vi "Analog Output - N Channels - N Samples.vi"() -> ()   [LabVIEW 2019]
uses:
  <vilib>/myRIO/Common/Instrument Driver Framework/ELVIS III v1.0/AO Block/vis/ELVIS III v1.0 Close AO Block.vi
  <vilib>/myRIO/Common/Instrument Driver Framework/myRIO v1.0/UART/vis/myRIO v1.0 Close UART.vi
  <vilib>/myRIO/Common/Instrument Driver Framework/ELVIS III v1.0/AO Block/vis/ELVIS III v1.0 Unreserve AO Block.vi
  <vilib>/myRIO/Common/Instrument Driver Framework/ELVIS III v1.0/AO Block/vis/ELVIS III v1.0 Build MUX Configuration AO Block.vi
  <vilib>/Utility/error.llb/Error Cluster From Error Code.vi
  <vilib>/myRIO/Common/Instrument Driver Framework/ELVIS III v1.0/AO Block/vis/ELVIS III v1.0 AO Block Write.vi
  <vilib>/myRIO/Common/Instrument Driver Framework/ELVIS III v1.0/Resource Manager/vis/ELVIS III v1.0 Unreserve Channel List.vi
  <vilib>/myRIO/Common/Instrument Driver Framework/myRIO v1.0/myRIO v1.0 Close.vi
  <vilib>/myRIO/Common/Instrument Driver Framework/Utilities/vis/FPGA Ref Manager.vi
  <vilib>/myRIO/Common/Instrument Driver Framework/ELVIS III v1.0/ELVIS III v1.0 Reset FPGA.vi
  <vilib>/myRIO/Common/Instrument Driver Framework/myRIO v1.0/IRQ/vis/myRIO v1.0 IRQ Info FGV.vi
  <vilib>/myRIO/Common/Instrument Driver Framework/myRIO v1.0/IRQ/vis/myRIO v1.0 Timer IRQ Info FGV.vi
  <vilib>/myRIO/Common/Instrument Driver Framework/myRIO v1.0/IRQ/vis/myRIO v1.0 ISR Agent.vi
  <vilib>/myRIO/Instrument Drivers/Utilities/vis/Reset Index.vi
  <vilib>/myRIO/Common/Instrument Driver Framework/myRIO v1.0/Resource Manager/vis/myRIO v1.0 Block Write Resource Manager.vi
  <vilib>/myRIO/Instrument Drivers/Utilities/Utilities.lvlib
  <vilib>/myRIO/Instrument Drivers/Onboard IO/AO Block/AO Block.lvlib
panel:
  in  "Generate Waveform":bool
  in  "AO1 - Triangle Frequency (Hz)":dbl=10.0 format="%#_13g"
  in  "AO1 - Triangle Amplitude (V)":dbl=5.0 min=-10.0 max=10.0 step=0.1 format="%#_13g"
  in  "AO0 - Sine Frequency (Hz)":dbl=10.0 format="%#_13g"
  in  "AO0 - Sine Amplitude (V)":dbl=5.0 min=-10.0 max=10.0 step=0.1 format="%#_13g"
  in  "Stop":bool
  # "ELVIS III Control IO"
  # "模拟输出N通道"
  # "Overview: Outputs one period of Sine and Triangle waves on Bank A, Channels AO0 and AO1 (A/AO0 and A/AO1).\nInstructions:\n1. Configure the sine wave and triangle wave properties below.\n2. Connect A/AO0 to the positive lead of a load, and connect AGND to the negative lead of the load. Connect A/AO1 to the positive lead of another load, and connect AGND to the negative lead of the corresponding load. AGND is the ground reference terminal for analog output channels.\n3. Run the VI.\n4. Modify the Amplitude and Frequency controls to change the sine and triangle waves.\n5. Press Generate Waveform to output the sine and triangle waves."
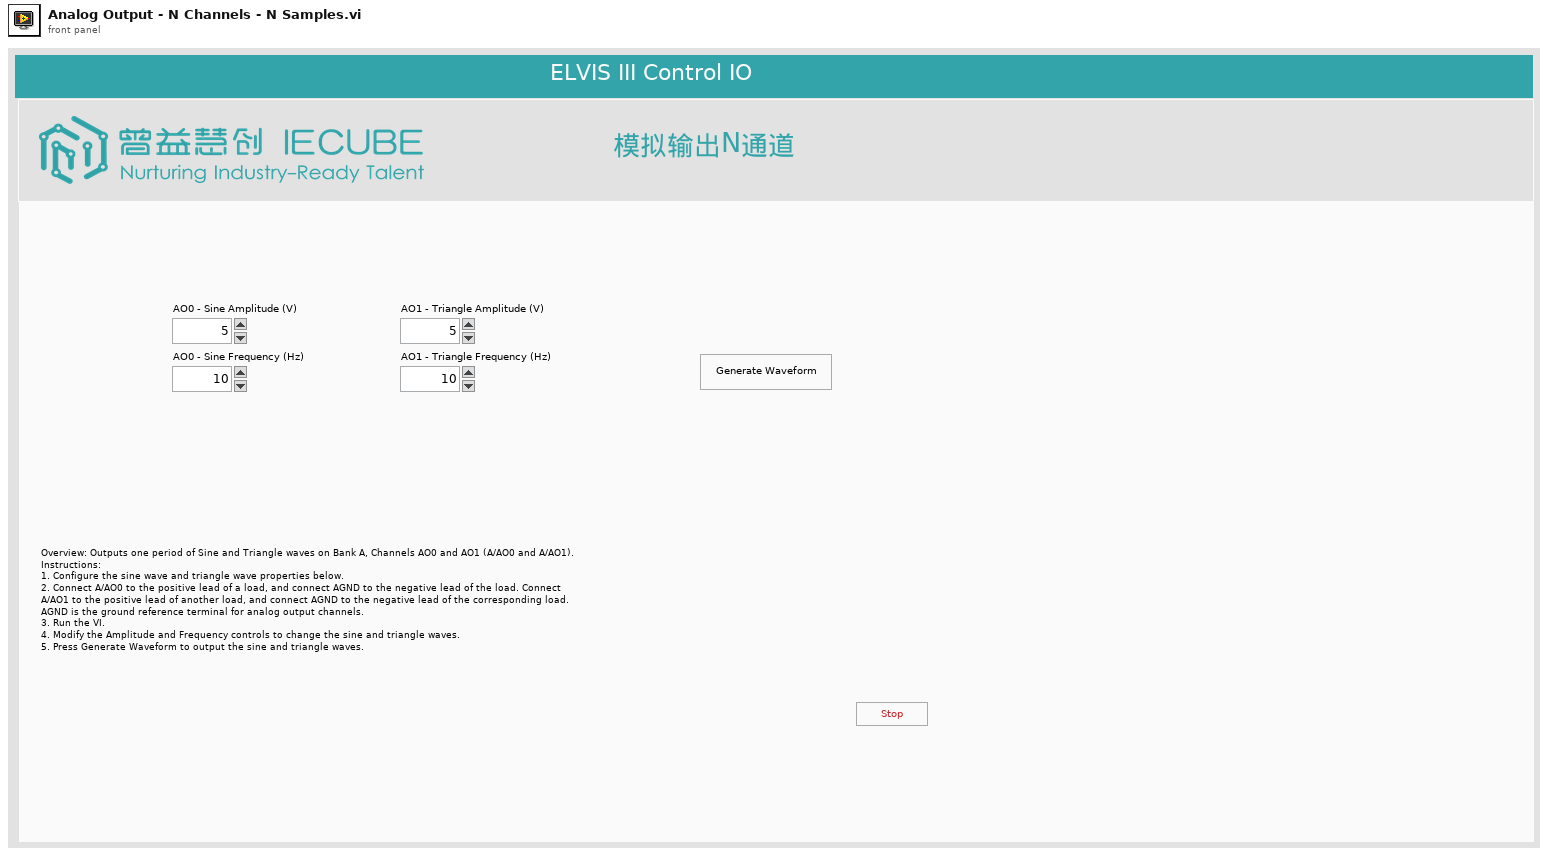
[diagram p1: front panel]
types:
  T1 = typedef "AO Block.lvlib/AO Block Reference.ctl" = cluster{"myRIO Reference":T2, "AO (N Samples) Channels List":T6, "AO (N Samples) Scaling Constants List":T8[]}
  T2 = typedef "myRIO Generic Hardware Reference.ctl" = cluster{"myRIO Model":T3, "myRIO Hardware Reference":T4}
  T3 = typedef "Hardware Version Enum.ctl" = enum16{"Unknown", "myRIO-1900", "myRIO-1950", "roboRIO", "NI ELVIS RIO CM", "ELVIS III"}
  T4 = typedef "myRIO v1.0 Reference.ctl" = cluster{"Generic FPGA Reference":T5, "Allow multiple opens":bool}
  T5 = typedef "Generic FPGA Reference.ctl" = refnum<k20>
  T6 = typedef "AO Block Channels List.ctl" = T7[]
  T7 = typedef "AO Block Channels Enum.ctl" = enum16{"Not Connected", "A/AO0 (N Samples)", "A/AO1 (N Samples)", "B/AO0 (N Samples)", "B/AO1 (N Samples)"}
  T8 = typedef "Analog Scaling Constants.ctl" = cluster{"LSB Weight (Volts)":dbl, "Offset (Volts)":dbl, "Signed?":bool}
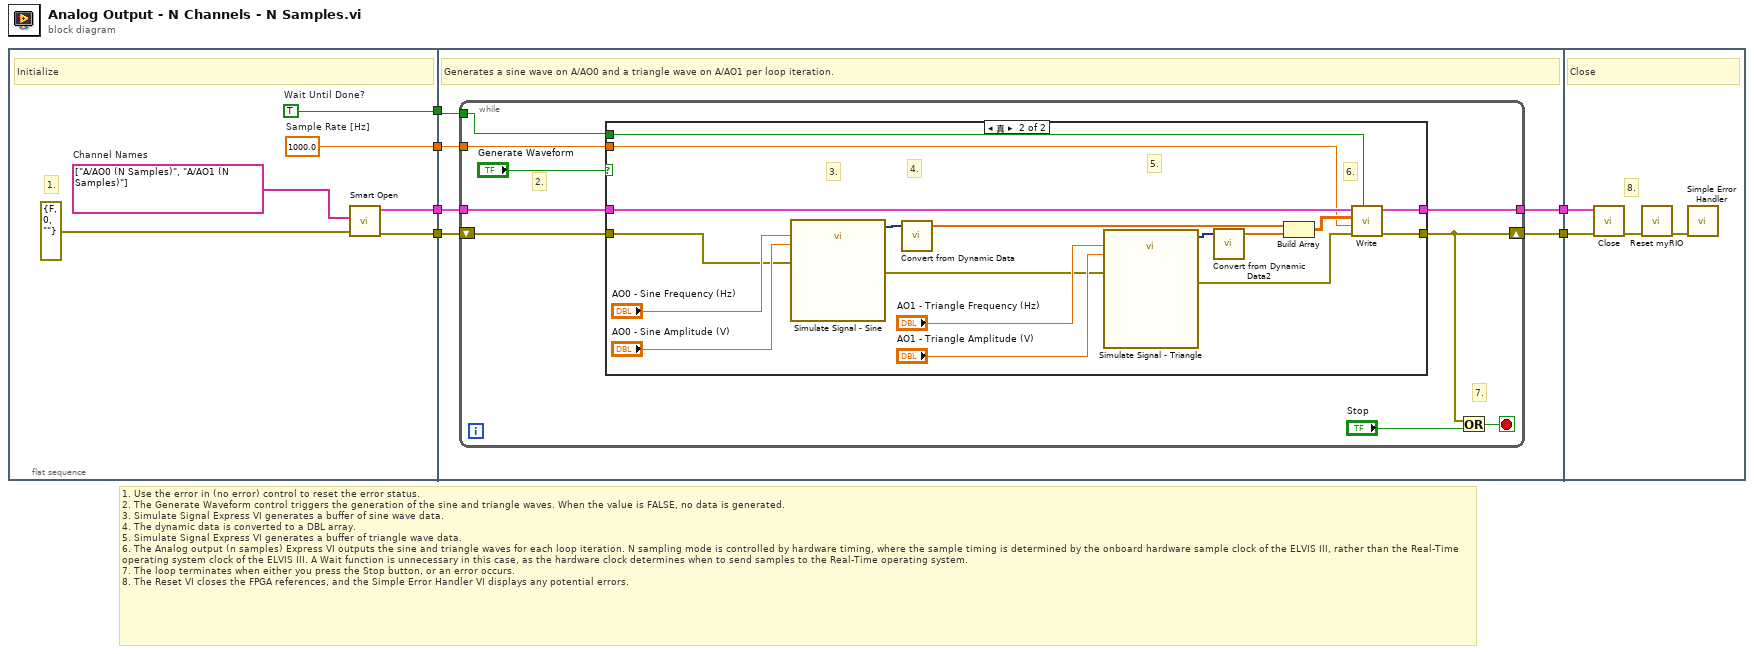
[diagram p0: block diagram]
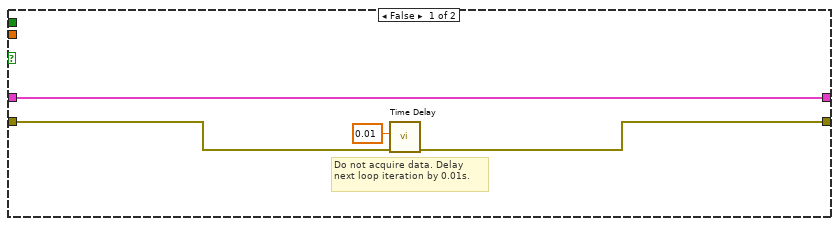
[diagram p2: hidden frame]
diagram:
  # "1. Use the error in (no error) control to reset the error status.\n2. The Generate Waveform control triggers the generation of the sine and triangle waves. When the value is FALSE, no data is generated.\n3. Simulate Signal Express VI generates a buffer of sine wave data.\n4. The dynamic data is converted to a DBL array.\n5. Simulate Signal Express VI generates a buffer of triangle wave data.\n6. The Analog output (n samples) Express VI outputs the sine and triangle waves for each loop iteration. N sampling mode is controlled by hardware timing, where the sample timing is determined by the onboard hardware sample clock of the ELVIS III, rather than the Real-Time operating system clock of the ELVIS III. A Wait function is unnecessary in this case, as the hardware clock determines when to send samples to the Real-Time operating system.\n7. The loop terminates when either you press the Stop button, or an error occurs.\n8. The Reset VI closes the FPGA references, and the Simple Error Handler VI displays any potential errors."
  n1 = flat-sequence {
    tunnel: [w10] -> w5
    tunnel: [w9] -> w4
    tunnel: [w8] -> w3
    tunnel: [w7] -> w2
    tunnel: [w18] -> w6
    tunnel: w5 -> [w17]
    tunnel: w4 -> [w16]
    tunnel: w3 -> [w14]
    tunnel: w2 -> [w15]
    tunnel: [w13] -> w1
    tunnel: w6 -> [w51]
    tunnel: w1 -> [w49]
    frame #0 {
      w8 = TRUE  # Wait Until Done?
      w7 = 1000.0  # Sample Rate [Hz]
      w12 = tag[] ["A/AO0 (N Samples)", "A/AO1 (N Samples)"]  # Channel Names
      # "1."
      # "Initialize"
      n2 = call <vilib>:"Smart Open.vi"("error in (no error)"=errorcluster {"status"=FALSE, "code"=0, "source"=""} ("Error In"), "Channel Names"=w12) -> ("error out"=w10:errorcluster, "AO (N Samples) Ref Out"=w9:T1)  [unwired: 8 in]
    }
    frame #1 {
      # "Generates a sine wave on A/AO0 and a triangle wave on A/AO1 per loop iteration."
      n3 = while {
        shift-right: [w26] -> w18
        shift-left: w17 -> [w24]
        tunnel: w16 -> [w22]
        tunnel: w15 -> [w20]
        tunnel: w14 -> [w21]
        tunnel: [w19] -> w13
        stop <- w27 stop-if-true
        # "2."
        # "7."
        n4 = case shown="真" "Generate Waveform" {
          tunnel: [w29 w38] -> w26
          tunnel: w24 -> [w30 w45]
          tunnel: w22 -> [w28 w35]
          tunnel: w21 -> [_ w33]
          tunnel: w20 -> [_ w34]
          tunnel: [w28 w32] -> w19
          frame False {
            # "Do not acquire data. Delay next loop iteration by 0.01s."
            n5 = call "Time Delay"("error in (no error)"=w30, "Delay Time (s)"=0.01) -> ("error out"=w29:errorcluster)  [unwired: 9 in]
          }
          frame True {
            # "6."
            # "5."
            # "4."
            # "3."
            n6 = call "Simulate Signal - Sine"("Frequency"="AO0 - Sine Frequency (Hz)", "Amplitude"="AO0 - Sine Amplitude (V)", "error in (no error)"=w45) -> ("Sine"=w46:dynamicdata, "error out"=w41:errorcluster)  [unwired: 11 in]
            n7 = call "Convert from Dynamic Data"("Dynamic Data Type"=w46) -> ("Array"=w37:dbl[])  [unwired: 3 in]
            n8 = call "Simulate Signal - Triangle"("Frequency"="AO1 - Triangle Frequency (Hz)", "Amplitude"="AO1 - Triangle Amplitude (V)", "error in (no error)"=w41) -> ("Triangle"=w44:dynamicdata, "error out"=w39:errorcluster)  [unwired: 11 in]
            n9 = call "Convert from Dynamic Data2"("Dynamic Data Type"=w44) -> ("Array"=w36:dbl[])  [unwired: 3 in]
            n10 = Build Array(w37, w36) -> (w40:dbl[][])
            n11 = call <vilib>:"Write.vi"("Wait Until Done?"=w33, "error in (no error)"=w39, "Sample Rate [Hz]"=w34, "Values"=w40, "AO (N Samples) Ref In"=w35) -> ("error out"=w38:errorcluster, "AO (N Samples) Ref Out"=w32:T1)  [unwired: 5 in]
          }
        }
        n12 = Or(x=w26, y="Stop") -> (x .or. y?=w27:bool)
      }
    }
    frame #2 {
      # "8."
      # "Close"
      n13 = call <vilib>:"Close.vi"("error in (no error)"=w51, "AO (N Samples) Ref In"=w49) -> ("error out"=w50:errorcluster)  [unwired: 9 in]
      n14 = call <vilib>:"Reset myRIO.vi"("error in (no error)"=w50) -> ("error out"=w52:errorcluster)  [unwired: 10 in]
      n15 = call <vilib>:"Simple Error Handler.vi"("error in (no error)"=w52) -> ()  [unwired: 4 in, 5 out]
    }
  }
